vi "Not a Num.vi"   [LabVIEW 2014]
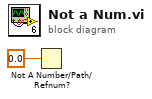
[diagram p0: block diagram]
diagram:
  n1 = Not A Number/Path/Refnum?(number/path/refnum=0.0 ("数字/路径/引用句柄")) -> ()  [unwired: 1 out]
